vi "Configure Waveform Sweep.vi"(8 "error in (no error)":errorcluster, 10 "Enable Waveform Sweep (F:Disable)":bool, 11 "VISA resource name":refnum<visa-resource-name>) -> (0 "error out":errorcluster, 3 "VISA resource name out":refnum<visa-resource-name>)   [LabVIEW 2012, in "Agilent PSG MXG Series.lvlib"]
doc: "Configures the waveform sweep function.\n\n<B>Notes:</B>\n(1) This VI is valid only in N5162A, N5182A, N5172B, N5182B.\n\n(2) For N5162A and N5182A, this VI is valid only when the instrument installs <B>Option 651</B> or <B>Option 652</B> or <B>Option 654</B> (Internal baseband generator)."
uses:
  <instrlib>/Agilent PSG MXG Series/Agilent PSG MXG Series.lvlib
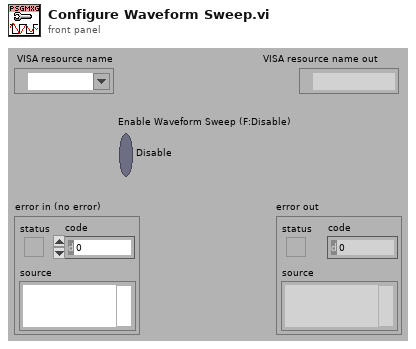
[diagram p1: front panel]
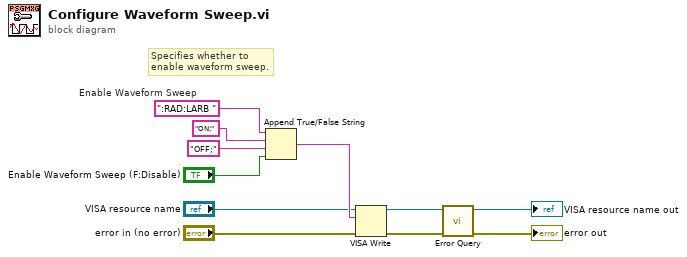
[diagram p0: block diagram]
diagram:
  w11 = ":RAD:LARB "  # Enable Waveform Sweep
  # "Specifies whether to\nenable waveform sweep."
  n1 = Append True/False String(1:"Enable Waveform Sweep (F:Disable)", 2:"OFF;" ("false string"), 3:"ON;" ("true string"), 4:w11) -> (0:w7:string)
  n2 = VISA Write(VISA resource name="VISA resource name", write buffer=w7, error in (no error)="error in (no error)") -> (VISA resource name out=w6:refnum<visa-resource-name>, error out=w5:errorcluster)  [unwired: 1 out]
  n3 = call <instrlib>:"Error Query.vi"("error in (no error)"=w5, "VISA resource name"=w6) -> ("error out"=→"error out":errorcluster, "VISA resource name out"=→"VISA resource name out":refnum<visa-resource-name>)  [unwired: 8 out]
